vi "Set External Phase Lock.vi"(8 "error in (no error)":errorcluster, 10 "External Phase Lock (F: Off)":bool, 11 "VISA resource name":refnum<visa-resource-name>) -> (0 "error out":errorcluster, 3 "VISA resource name out":refnum<visa-resource-name>)   [LabVIEW 2013, in "Fluke 5XXX Series Multicalibrators.lvlib"]
doc: "This VI enables or disables external phase locking, when the calibrator is supplying an ac voltage.\n\nNote:\n\nThis VI is available only for instrument models 5700A and 5720A."
uses:
  Fluke 5XXX Series Multicalibrators.lvlib
panel:
  # "On"
  # "Off"
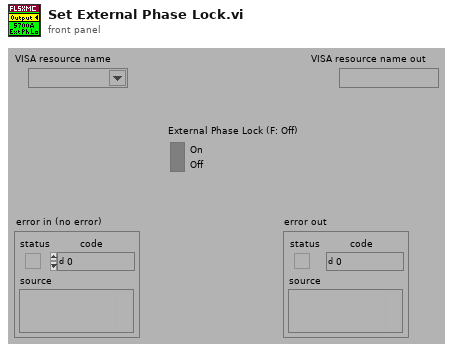
[diagram p1: front panel]
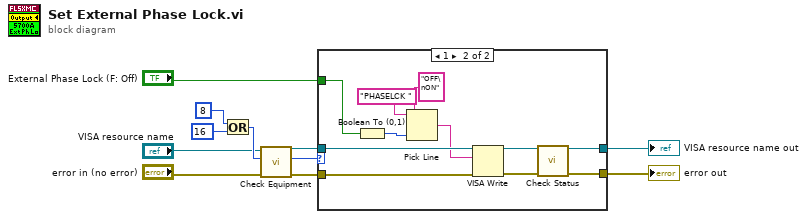
[diagram p0: block diagram]
diagram:
  n1 = Or(x=8 ("Numeric"), y=16 ("Numeric")) -> (x .or. y?=w7:i32)
  n2 = call "Check Equipment.vi"("error in (no error)"="error in (no error)", "Bit Mask"=w7, "VISA resource name"="VISA resource name") -> ("error out"=w11:errorcluster, "Present?"=w10:u32, "VISA resource name out"=w9:refnum<visa-resource-name>)  [unwired: 6 in]
  n3 = case shown="1" w10 {
    tunnel: "External Phase Lock (F: Off)" -> [_ w21]
    tunnel: [w12 w15] -> w1
    tunnel: w11 -> [w13 w20]
    tunnel: w9 -> [w12 w19]
    tunnel: [w13 w16] -> w2
    frame 0, Default {
    }
    frame 1 {
      n4 = Boolean To (0,1)(Boolean=w21) -> (0, 1=w22:i16)
      n5 = Pick Line(string ("")="PHASELCK " ("Reset Command"), multi-line string="OFF\nON", line index=w22) -> (output string=w18:string)
      n6 = VISA Write(VISA resource name=w19, write buffer=w18, error in (no error)=w20) -> (VISA resource name out=w14:refnum<visa-resource-name>, error out=w17:errorcluster)  [unwired: 1 out]
      n7 = call "Check Status.vi"("VISA resource name"=w14, "error in (no error)"=w17) -> ("VISA resource name out"=w15:refnum<visa-resource-name>, "error out"=w16:errorcluster)  [unwired: 12 in]
    }
  }
  "VISA resource name out" <- w1
  "error out" <- w2
